vi "Fault List with Timer.vi"(8 "error in (no error)":errorcluster, 10 "Delay":dbl=15.0) -> (0 "error out":errorcluster, 2 "Fault Strings":string[](array[string]), 3 "Faults Present":bool)   [LabVIEW 2009]
uses:
  Faults List Actions.ctl
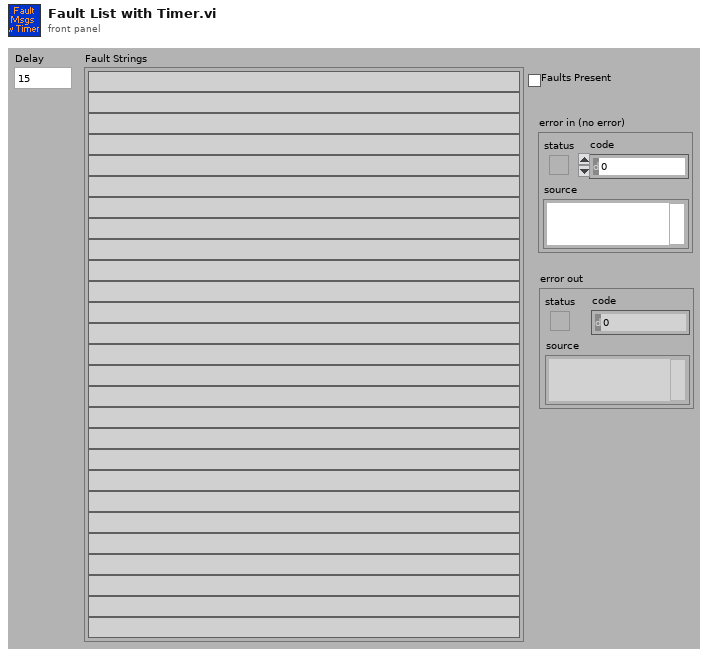
[diagram p1: front panel]
types:
  T1 = typedef "Faults List Actions.ctl" = enum16{"Init", "Add", "Remove", "Get List"}
  T2 = typedef "Fault Id.ctl" = cluster{"Fault Type":T3, "LBCB Number":T4, "Index":u32, "Space Type":T5}
  T3 = typedef "Fault Type.ctl" = enum16{"None", "Command", "Displacement", "Force", "Increment"}
  T4 = typedef "LBCB Number.ctl" = enum16{"LBCB1", "LBCB2"}
  T5 = typedef "Space Type.ctl" = enum16{"Actuator", "Cartesian"}
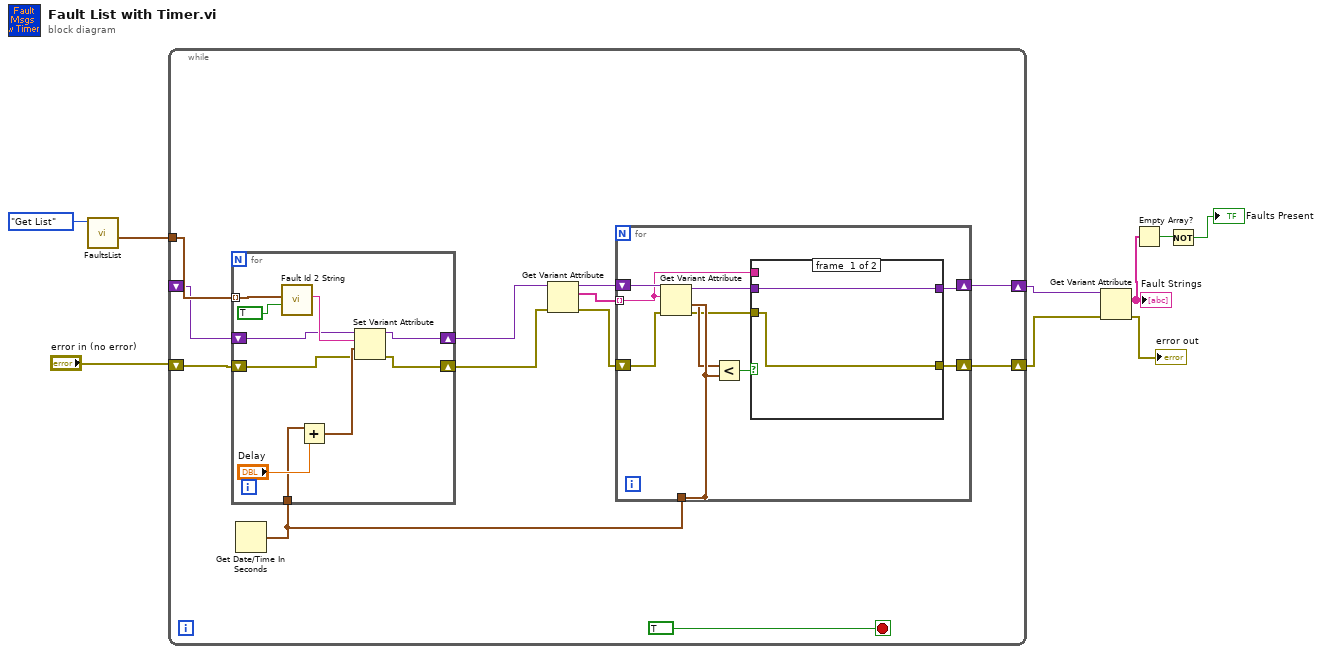
[diagram p0: block diagram]
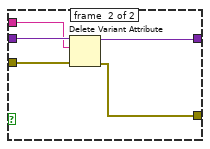
[diagram p2: hidden frame]
diagram:
  n1 = call "FaultsList.vi"("Limits List Actions"=Faults_List_Actions."Get List") -> ("Fault List"=w8:T2[])  [unwired: 2 in, 8 out]
  n2 = while {
    shift-right: [w15] -> w7
    shift-left: _ -> [w19]
    tunnel: w8 -> [w20]
    shift-right: [w12] -> w6
    shift-left: "error in (no error)" -> [w18]
    stop <- TRUE stop-if-true
    n3 = Get Date/Time In Seconds() -> (seconds since 1Jan1904=w11:timestamp)
    n4 = for {
      tunnel: w20 -> [w48] mode=indexing
      shift-right: [w46] -> w16
      shift-left: w19 -> [w44]
      shift-right: [w40] -> w14
      shift-left: w18 -> [w41]
      tunnel: w11 -> [w39]
      n5 = call "Fault Id 2 String.vi"("Add LBCB Type"=TRUE, "Fault Id In"=w48) -> ("String"=w45:string)  [unwired: 9 in]
      n6 = Add(x=w39, y="Delay") -> (x+y=w42:timestamp)
      n7 = Set Variant Attribute(Variant=w44, name=w45, value=w42, error in=w41) -> (Variant out=w46:variant, error out=w40:errorcluster)  [unwired: 1 out]
    }
    n8 = Get Variant Attribute(Variant=w16, error in=w14) -> (duplicate Variant=w10:variant, names=w17:string[], error out=w13:errorcluster)  [unwired: 2 in, 1 out]
    n9 = for {
      tunnel: w17 -> [w25] mode=indexing
      shift-right: [w26] -> w15
      shift-left: w10 -> [w31]
      shift-right: [w22] -> w12
      shift-left: w13 -> [w24]
      tunnel: [w30] -> _
      tunnel: w11 -> [w30]
      n10 = Get Variant Attribute(Variant=w31, name=w25, default value (empty Variant)=w30, error in=w24) -> (duplicate Variant=w27:variant, value=w29:timestamp, error out=w23:errorcluster)  [unwired: 1 out]
      n11 = Less?(x=w29, y=w30) -> (x < y?=w28:bool)
      n12 = case shown="True" w28 {
        tunnel: w27 -> [w33 w38]
        tunnel: [w33 w34] -> w26
        tunnel: w25 -> [_ w37]
        tunnel: w23 -> [w32 w36]
        tunnel: [w32 w35] -> w22
        frame #0 {
        }
        frame #1 {
          n13 = Delete Variant Attribute(4:w36, 6:w37, 7:w38) -> (0:w35:errorcluster, 3:w34:variant)  [unwired: 1 out]
        }
      }
    }
  }
  n14 = Get Variant Attribute(Variant=w7, error in=w6) -> (names=w3:string[], error out=→"error out":errorcluster)  [unwired: 2 in, 2 out]
  "Fault Strings" <- w3
  n15 = Empty Array?(array=w3) -> (empty?=w2:bool)
  n16 = Not(x=w2) -> (.not. x?=→"Faults Present":bool)
